vi "Init.vi"(6 "Connection":refnum<class "Connection.lvclass">, 8 "error in (no error)":errorcluster, 9 "Out Count":i32, 10 "In Count":i32) -> (0 "error out":errorcluster, 3 "Mux out":refnum<class "Mux.lvclass">)   [LabVIEW 2022 SP3, in "VideoMux.lvlib" / "Mux.lvclass"]
uses:
  Mux.lvclass
  <vilib>/IlluminatedG/lv-stream/Connection/Connection.lvclass
  Mux.lvclass/Mux.ctl
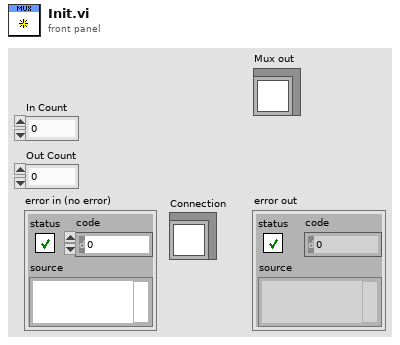
[diagram p1: front panel]
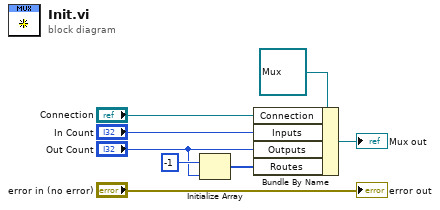
[diagram p0: block diagram]
diagram:
  n1 = Initialize Array(-1, "Out Count") -> (w7:i32[])
  n2 = Bundle By Name(cluster=refnum<class "Mux.lvclass"> refnum ("Mux in"), "Connection"="Connection", "Inputs"="In Count", "Outputs"="Out Count", "Routes"=w7) -> (→"Mux out":refnum<class "Mux.lvclass">)
  "error out" <- "error in (no error)"
